vi "Rec_organize data.vi"(7 "only Z":bool, 9 "beads track":T1[](array[typedef]) {"centroid"."Y Centroid" format="%.2f"; "centroid"."X Centroid" format="%.2f"; "ROI Des out"."Contours"."Type" items=["No Selection", "Point", "Line", "Rectangle", "Oval", "Polygon", "Freehand Region", "Annulus", "Unused2", "Unused3", "Broken Line", "Freehand Line", "Rotated Rectangle"]}) -> (2 "rec array":dbl[][][](array[numeric]), 3 "Array":string[](array[string]))   [LabVIEW 2017]
doc: "本VI的作用是将分析循环得出的XYZ信息，以及当前的磁铁位置信息，按照磁球序号进行重新组织，方便写入TDMS文件，组织顺序和创建的通道顺序一致。\n组织过程中可以选取一个磁球作为参考球，但也可以选择不要参考球。"
uses:
  control/Bead track.ctl
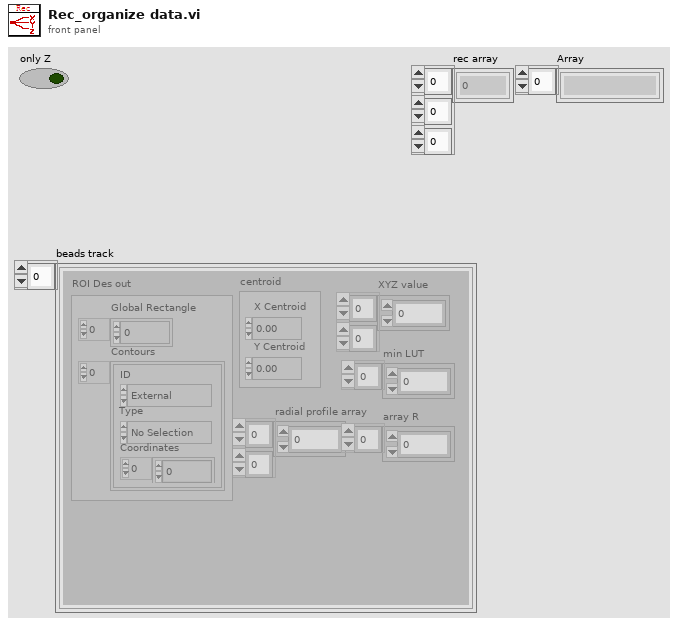
[diagram p1: front panel]
types:
  T1 = typedef "Bead track.ctl" = cluster{"XYZ value":dbl[][], "radial profile array":dbl[][], "min LUT":dbl[], "ROI Des out":T2, "array R":dbl[], "centroid":cluster{"X Centroid":sgl, "Y Centroid":sgl}}
  T2 = typedef "ROI Descriptor" = cluster{"Global Rectangle":i32[], "Contours":cluster{"ID":enum32{"External", "Internal"}, "Type":u32, "Coordinates":i32[]}[]}
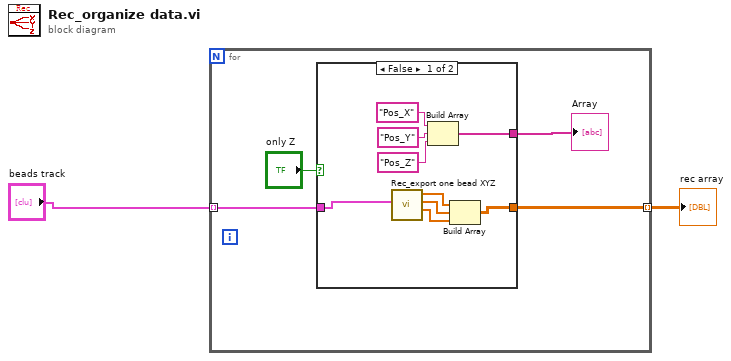
[diagram p0: block diagram]
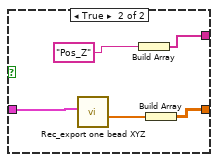
[diagram p2: hidden frame]
diagram:
  n1 = for {
    tunnel: "beads track" -> [w6] mode=indexing
    tunnel: [w5] -> w1 mode=indexing
    n2 = case shown="False" "only Z" {
      tunnel: w6 -> [w15 w20]
      tunnel: [w11 w19] -> w5
      tunnel: [w7 w16] -> w3
      frame False {
        n3 = call "Rec_export one bead XYZ.vi"("beads track"=w15) -> ("Z"=w14:dbl[], "Y"=w13:dbl[], "X"=w12:dbl[])  [unwired: 8 in]
        n4 = Build Array("Pos_X" ("字符串"), "Pos_Y" ("字符串"), "Pos_Z" ("字符串")) -> (w7:string[])
        n5 = Build Array(w12, w13, w14) -> (w11:dbl[][])
      }
      frame True {
        n6 = call "Rec_export one bead XYZ.vi"("beads track"=w20) -> ("Z"=w18:dbl[])  [unwired: 8 in, 2 out]
        n7 = Build Array("Pos_Z" ("字符串")) -> (w16:string[])
        n8 = Build Array(w18) -> (w19:dbl[][])
      }
    }
    "Array" <- w3
  }
  "rec array" <- w1
